vi "Create Empty Waveform Array.vi"(8 "error in (no error)":errorcluster caption="错误输入（无错误）", 10 "Acquisition Info":T1 caption="数采信息", 11 "Timestamp":timestamp caption="时间标识") -> (0 "error out":errorcluster caption="错误输出", 3 "Waveform Array":waveform(dbl)[](array[waveform]) caption="波形数据")   [LabVIEW 2015]
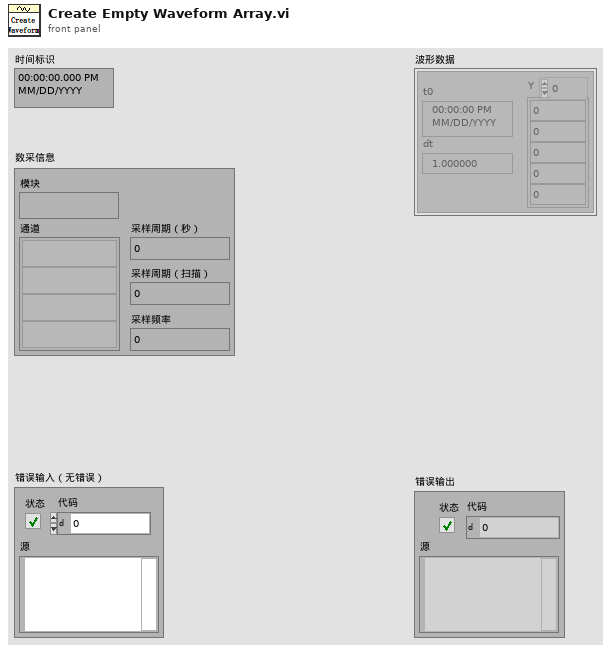
[diagram p1: front panel]
types:
  T1 = cluster{"Module":string, "Channels":string[], "Sampling Period(S)":dbl, "Sampling Period(Scan)":i64, "Sampling Frequency":i32}
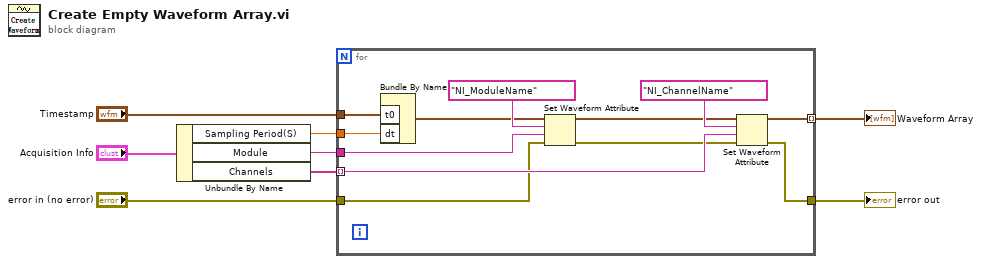
[diagram p0: block diagram]
diagram:
  n1 = Unbundle By Name("Acquisition Info") -> ("Sampling Period(S)"=w6:dbl, "Module"=w7:string, "Channels"=w8:string[])
  n2 = for {
    tunnel: "Timestamp" -> [w20]
    tunnel: w6 -> [w16]
    tunnel: w7 -> [w19]
    tunnel: w8 -> [w18] mode=indexing
    tunnel: [w17] -> w2 mode=indexing
    tunnel: "error in (no error)" -> [w15]
    tunnel: [w13] -> w3
    n3 = Bundle By Name("t0"=w20, "dt"=w16) -> (w10:waveform(dbl))  [unwired: 1 in]
    n4 = Set Waveform Attribute(4:w15, 5:w19, 6:"NI_ModuleName", 7:w10) -> (0:w14:errorcluster, 3:w9:waveform(dbl))  [unwired: 1 out]
    n5 = Set Waveform Attribute(4:w14, 5:w18, 6:"NI_ChannelName", 7:w9) -> (0:w13:errorcluster, 3:w17:waveform(dbl))  [unwired: 1 out]
  }
  "error out" <- w3
  "Waveform Array" <- w2
